vi "tracking1.vi"(6 "lane keep":bool, 10 "xbody":dbl, 11 "xt":dbl) -> (3 "handle":dbl=-3.32529799262397, 5 "Numeric":i32)   [LabVIEW 2015]
uses:
  G_PATH.vi
  G_VEH.vi
  G_NAV.vi
  G_SEN.vi
panel:
  out "v250":dbl[](array[numeric]) format="%.2f"
  in  "gain":dbl=0.7000000000000001
  in  "x":dbl=10.0
  in  "y":dbl=42.0
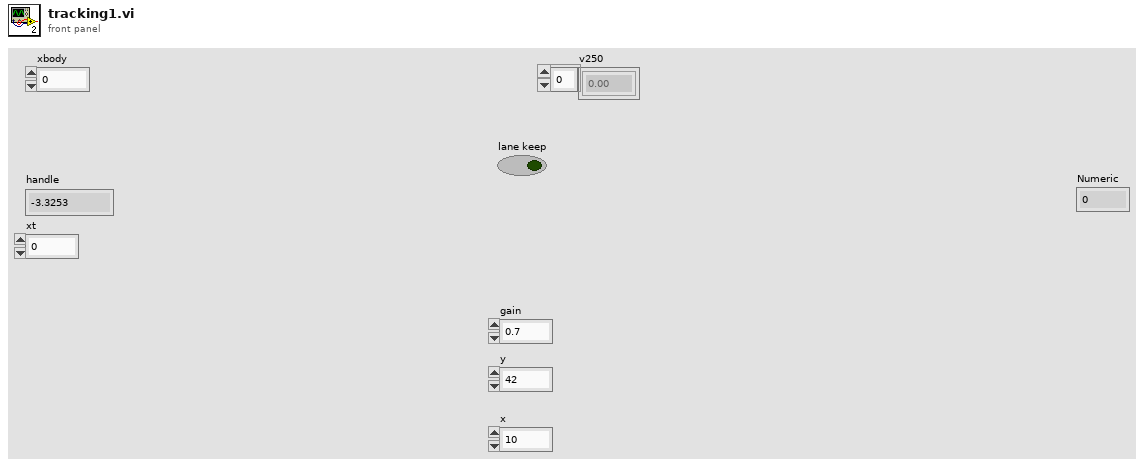
[diagram p1: front panel]
types:
  T1 = cluster{"idx":i32, "x":dbl, "y":dbl, "h":dbl, "x_path":dbl}
  T2 = cluster{"Steer_input":dbl, "Steer_output":dbl, "VS_des":dbl, "VS_can":dbl, "heading":dbl, "auto":bool, "run":bool, "x":dbl, "y":dbl}
  T3 = cluster{"GPSTime":dbl, "attitude[2]":dbl, "lcc[0]":dbl, "lcc[1]":dbl, "heading_GPS":dbl}
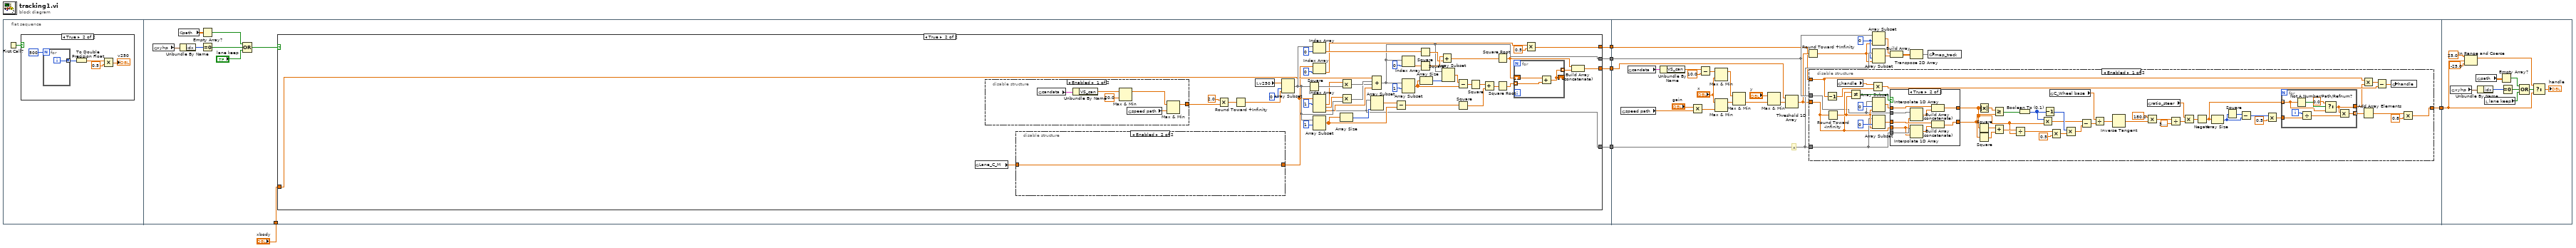
[diagram p0: block diagram]
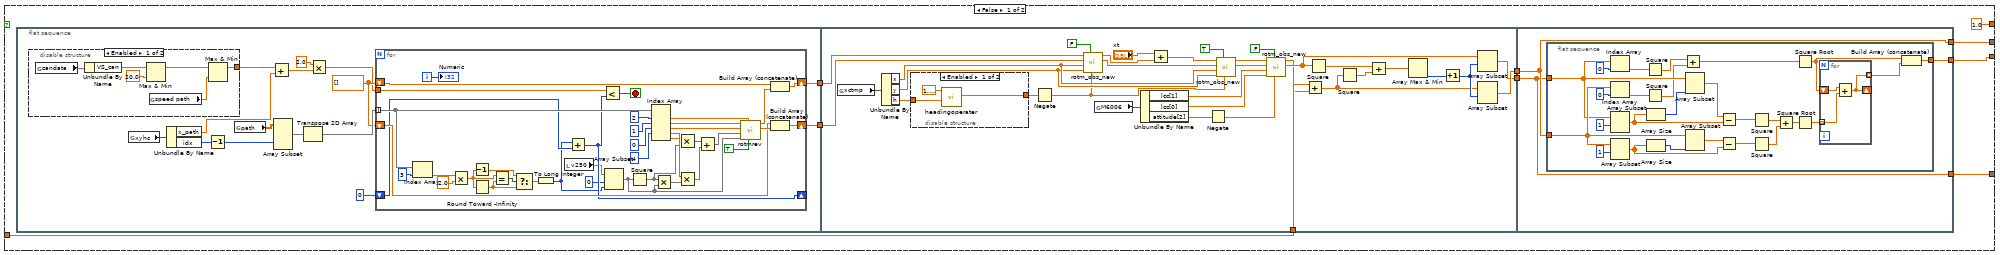
[diagram p3: hidden frame]
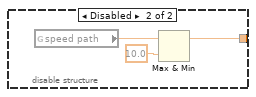
[diagram p4: hidden frame]
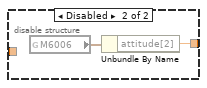
[diagram p5: hidden frame]
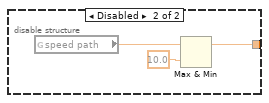
[diagram p6: hidden frame]
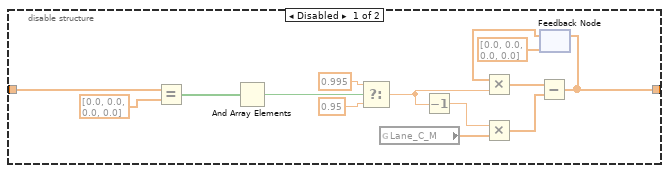
[diagram p7: hidden frame]
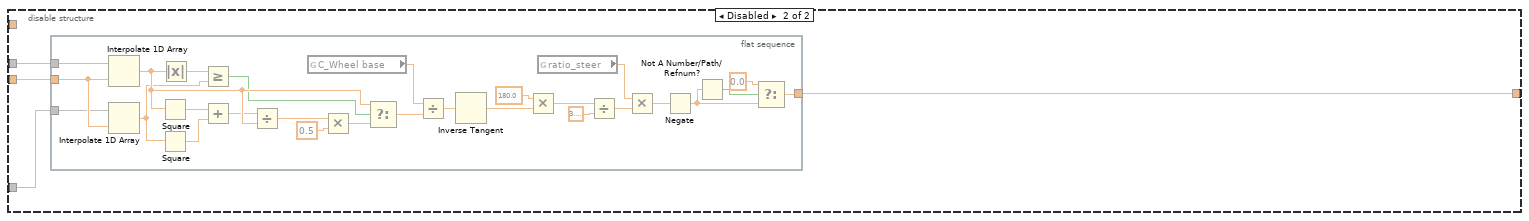
[diagram p9: hidden frame]
diagram:
  n1 = flat-sequence {
    tunnel: [w25] -> w6
    tunnel: [w24] -> w5
    tunnel: [w23] -> w4
    tunnel: "xbody" -> [w15]
    tunnel: [w14] -> w1
    tunnel: w6 -> [w262]
    tunnel: w5 -> [w252]
    tunnel: w4 -> [w251]
    tunnel: [w248] -> w3
    tunnel: w1 -> [w245]
    tunnel: w3 -> [w366]
    frame #0 {
      n2 = First Call?() -> (First Call?: T/F=w7:bool)
      n3 = case shown="True" w7 {
        frame False {
        }
        frame True {
          n4 = for {
            N: 500 -> [_]
            tunnel: [w13] -> w9 mode=indexing
            i -> [w13]
          }
          n5 = To Double Precision Float(number=w9) -> (double precision float=w10:dbl[])
          n6 = Multiply(x=w10, y=0.5 ("x")) -> (x*y=→"v250":dbl[])
        }
      }
    }
    frame #1 {
      n7 = global read "G_VEH.vi" "xyhp"() -> (w21:T1)
      n8 = global read "G_PATH.vi" "path"() -> (w18:dbl[][])
      n9 = Unbundle By Name(w21) -> ("idx"=w20:i32)
      n10 = Empty Array?(array=w18) -> (empty?=w17:bool)
      n11 = Equal To 0?(x=w20) -> (x = 0?=w19:bool)
      n12 = Compound Arithmetic op=OR(w17, w19, "lane keep") -> (w16:bool)
      n13 = case shown="True" w16 {
        tunnel: [w30 w204] -> w25
        tunnel: [w29 w180] -> w24
        tunnel: [w28 w174] -> w23
        tunnel: w15 -> [w27 w173]
        tunnel: [1.0 w168] -> w14
        frame False {
          n14 = flat-sequence {
            tunnel: [w42] -> w34
            tunnel: [w41] -> w33
            tunnel: [w124] -> w32
            tunnel: [w123] -> w31
            tunnel: w34 -> [w126]
            tunnel: w33 -> [w125]
            tunnel: w27 -> [w100]
            tunnel: w32 -> [w137]
            tunnel: w31 -> [w136]
            tunnel: [w138] -> w30
            tunnel: [w137] -> w29
            tunnel: [w136] -> w28
            frame #0 {
              w43 = dbl[] []
              n15 = disable-structure shown="Enabled" {
                disable-tunnel: [w50 w56] -> w35
                frame Enabled {
                  n16 = global read "G_VEH.vi" "candata"() -> (w55:T2)
                  n17 = Unbundle By Name(w55) -> ("VS_can"=w54:dbl)
                  n18 = Max & Min(x=w54, y=20.0) -> (max(x,y)=w52:dbl)  [unwired: 1 out]
                  n19 = global read "G_VEH.vi" "speed path"() -> (w51:dbl)
                  n20 = Max & Min(x=w52, y=w51) -> (max(x,y)=w50:dbl)  [unwired: 1 out]
                }
                frame Disabled {
                  n21 = global read "G_VEH.vi" "speed path"() -> (w58:dbl)
                  n22 = Max & Min(x=w58, y=10.0) -> (max(x,y)=w56:dbl)  [unwired: 1 out]
                }
              }
              n23 = global read "G_VEH.vi" "xyhc"() -> (w49:T1)
              n24 = Unbundle By Name(w49) -> ("x_path"=w36:dbl, "idx"=w48:i32)
              n25 = Decrement(x=w48) -> (x-1=w47:i32)
              n26 = global read "G_PATH.vi" "path"() -> (w46:dbl[][])
              n27 = Add(x=w35, y=w36) -> (x+y=w40:dbl)
              n28 = Array Subset(array=w46, index (col)=w47) -> (w45:dbl[][])  [unwired: 3 in]
              n29 = Transpose 2D Array(2D array=w45) -> (transposed array=w44:dbl[][])
              n30 = Multiply(x=2.0, y=w40) -> (x*y=w38:dbl)
              n31 = for {
                tunnel: w44 -> [w74] mode=indexing
                shift-right: [w72] -> w42
                shift-left: w43 -> [w71]
                shift-right: [w69] -> w41
                shift-left: w43 -> [w68]
                tunnel: w38 -> [w66]
                shift-right: [w65] -> _
                shift-left: 0 -> [w67]
                i -> [w64]
                stop <- w63 stop-if-true
                n32 = Index Array(array=w74, index=3) -> (element=w96:dbl)
                n33 = Multiply(x=w96, y=2.0) -> (x*y=w94:dbl)
                n34 = Decrement(x=w94) -> (x-1=w92:dbl)
                n35 = Round Toward -Infinity(1:w94) -> (0:w91:dbl)
                n36 = Equal?(x=w94, y=w91) -> (x = y?=w93:bool)
                n37 = Select(t=w92, s=w93, f=w91) -> (s? t:f=w90:dbl)
                n38 = To Long Integer(number=w90) -> (32bit integer=w60:i32)
                n39 = local read "v250"() -> (w62:dbl[])
                n40 = Add(x=w60, y=w67) -> (x+y=w65:i32)
                n41 = Less?(x=w66, y=w65) -> (x < y?=w63:bool)
                n42 = Array Subset(array=w62, index=0, length=w60) -> (w59:dbl[])
                n43 = Square(x=w59) -> (x^2=w77:dbl[])
                n44 = Index Array(array=w74, index #1=2 ("index"), index #2=1 ("index"), index #3=0 ("index"), index #4=4 ("index")) -> (element #1=w86:dbl, element #2=w87:dbl, element #3=w88:dbl, element #4=w78:dbl, element #5=w76:dbl)  [unwired: 1 in]
                n45 = Multiply(x=w77, y=w59) -> (x*y=w79:dbl[])
                n46 = Multiply(x=w76, y=w77) -> (x*y=w80:dbl[])
                n47 = Multiply(x=w78, y=w79) -> (x*y=w81:dbl[])
                n48 = Add(x=w80, y=w81) -> (x+y=w82:dbl[])
                n49 = call "rotmrev.vi"("reverse"=TRUE, "angle[rad]"=w86, "x"=w59, "y"=w82, "x0"=w88, "y0"=w87) -> ("y"=w70:dbl[], "x"=w73:dbl[])  [unwired: 4 in]
                n50 = Build Array (concatenate)(w71, w73) -> (w72:dbl[])
                n51 = Build Array (concatenate)(w68, w70) -> (w69:dbl[])
                "Numeric" <- w64
              }
            }
            frame #1 {
              n52 = global read "G_VEH.vi" "xctmp"() -> (w129:T1)
              n53 = Unbundle By Name(w129) -> ("x"=w112:dbl, "y"=w111:dbl, "h"=w128:dbl)
              n54 = disable-structure shown="Enabled" {
                disable-tunnel: w128 -> [w132 _]
                disable-tunnel: [w131 w134] -> w120
                frame Enabled {
                  n55 = call "headingoperater.vi"("h1"=w132, "h2"=1.5707963267948966) -> ("h2-h1"=w131:dbl)  [unwired: 8 in, 1 out]
                }
                frame Disabled {
                  n56 = global read "G_NAV.vi" "M6006"() -> (w135:T3)
                  n57 = Unbundle By Name(w135) -> ("attitude[2]"=w134:dbl)
                }
              }
              n58 = Negate(x=w120) -> (-x=w110:dbl)
              n59 = call "rotm_obs_new.vi"("angle[rad]"=w110, "reverse"=FALSE, "y0"=w111, "x0"=w112, "y"=w125, "x"=w126) -> ("rot*(y-y0) 2"=w114:dbl[], "rot*(x-x0)"=w119:dbl[])  [unwired: 2 in, 2 out]
              n60 = global read "G_NAV.vi" "M6006"() -> (w107:T3)
              n61 = Unbundle By Name(w107) -> ("lcc[1]"=w106:dbl, "lcc[0]"=w105:dbl, "attitude[2]"=w102:dbl)
              n62 = Add(x="xt", y=w119) -> (x+y=w115:dbl[])
              n63 = Negate(x=w102) -> (-x=w101:dbl)
              n64 = call "rotm_obs_new.vi"("angle[rad]"=w110, "reverse"=TRUE, "y0"=w111, "x0"=w112, "y"=w114, "x"=w115) -> ("rot*(y-y0) 2"=w108:dbl[], "rot*(x-x0)"=w109:dbl[])  [unwired: 2 in, 2 out]
              n65 = call "rotm_obs_new.vi"("angle[rad]"=w101, "reverse"=FALSE, "y0"=w105, "x0"=w106, "y"=w108, "x"=w109) -> ("rot*(y-y0) 2"=w103:dbl[], "rot*(x-x0)"=w98:dbl[])  [unwired: 2 in, 2 out]
              n66 = Add(x=w100, y=w98) -> (x+y=w99:dbl[])
              n67 = Square(x=w103) -> (x^2=w117:dbl[])
              n68 = Square(x=w99) -> (x^2=w116:dbl[])
              n69 = Add(x=w117, y=w116) -> (x+y=w127:dbl[])
              n70 = Array Max & Min(array=w127) -> (min index (indices)=w122:i32)  [unwired: 3 out]
              n71 = Increment(x=w122) -> (x+1=w121:i32)
              n72 = Array Subset(array=w103, index=w121) -> (w123:dbl[])  [unwired: 1 in]
              n73 = Array Subset(array=w99, index=w121) -> (w124:dbl[])  [unwired: 1 in]
            }
            frame #2 {
              n74 = flat-sequence {
                tunnel: [w145] -> w138
                tunnel: w137 -> [w144]
                tunnel: w136 -> [w143]
                frame #0 {
                  n75 = Index Array(array=w143, index=0) -> (element=w148:dbl)
                  n76 = Index Array(array=w144, index=0) -> (element=w149:dbl)
                  n77 = Array Subset(array=w143, index=1) -> (w158:dbl[])  [unwired: 1 in]
                  n78 = Array Subset(array=w144, index=1) -> (w161:dbl[])  [unwired: 1 in]
                  n79 = Square(x=w148) -> (x^2=w140:dbl)
                  n80 = Square(x=w149) -> (x^2=w139:dbl)
                  n81 = Array Size(array=w158) -> (size(s)=w156:i32)
                  n82 = Array Size(array=w161) -> (size(s)=w163:i32)
                  n83 = Add(x=w140, y=w139) -> (x+y=w147:dbl)
                  n84 = Array Subset(array=w143, length=w156) -> (w157:dbl[])  [unwired: 1 in]
                  n85 = Array Subset(array=w144, length=w163) -> (w162:dbl[])  [unwired: 1 in]
                  n86 = Subtract(x=w157, y=w158) -> (x-y=w159:dbl[])
                  n87 = Subtract(x=w162, y=w161) -> (x-y=w160:dbl[])
                  n88 = Square(x=w159) -> (x^2=w141:dbl[])
                  n89 = Square(x=w160) -> (x^2=w142:dbl[])
                  n90 = Add(x=w141, y=w142) -> (x+y=w153:dbl[])
                  n91 = Square Root(x=w147) -> (sqrt(x)=w146:dbl)
                  n92 = Square Root(x=w153) -> (sqrt(x)=w152:dbl[])
                  n93 = for {
                    tunnel: w152 -> [w166] mode=indexing
                    shift-right: [w165] -> _
                    shift-left: w146 -> [w167]
                    tunnel: [w165] -> w154 mode=indexing
                    n94 = Add(x=w167, y=w166) -> (x+y=w165:dbl)
                  }
                  n95 = Build Array (concatenate)(w146, w154) -> (w145:dbl[])
                }
              }
            }
          }
        }
        frame True {
          n96 = global read "G_SEN.vi" "Lane_C_M"() -> (w179:dbl[])
          n97 = disable-structure shown="Enabled" {
            disable-tunnel: [w214 w220] -> w178
            frame Enabled {
              n98 = global read "G_VEH.vi" "candata"() -> (w219:T2)
              n99 = Unbundle By Name(w219) -> ("VS_can"=w218:dbl)
              n100 = Max & Min(x=w218, y=20.0) -> (max(x,y)=w216:dbl)  [unwired: 1 out]
              n101 = global read "G_VEH.vi" "speed path"() -> (w215:dbl)
              n102 = Max & Min(x=w216, y=w215) -> (max(x,y)=w214:dbl)  [unwired: 1 out]
            }
            frame Disabled {
              n103 = global read "G_VEH.vi" "speed path"() -> (w222:dbl)
              n104 = Max & Min(x=w222, y=10.0) -> (max(x,y)=w220:dbl)  [unwired: 1 out]
            }
          }
          n105 = disable-structure shown="Enabled" {
            disable-tunnel: [w233 w237] -> w172
            disable-tunnel: w179 -> [w228 w237]
            frame Disabled {
              n106 = Equal?(x=w228, y=dbl[] [0.0, 0.0, 0.0, 0.0] ("Lane_C_M")) -> (x = y?=w227:bool[])
              n107 = And Array Elements(Boolean array=w227) -> (logical AND=w226:bool)
              n108 = Select(t=0.995, s=w226, f=0.95 ("filter")) -> (s? t:f=w225:dbl)
              n109 = global read "G_SEN.vi" "Lane_C_M"() -> (w230:dbl[])
              n110 = Decrement(x=w225) -> (x-1=w231:dbl)
              n111 = Multiply(x=w231, y=w230) -> (x*y=w236:dbl[])
              n112 = feedback #1(dbl[] [0.0, 0.0, 0.0, 0.0] ("Lane_C_M")) -> (w235:dbl[])
              n113 = Multiply(x=w235, y=w225) -> (x*y=w234:dbl[])
              n114 = Subtract(x=w234, y=w236) -> (x-y=w233:dbl[])
              n115 = feedback-in #1(w233) -> ()
            }
            frame Enabled {
            }
          }
          n116 = Multiply(x=2.0, y=w178) -> (x*y=w212:dbl)
          n117 = Round Toward +Infinity(x=w212) -> (ceil(x): smallest int >= x=w176:dbl)
          n118 = local read "v250"() -> (w177:dbl[])
          n119 = Array Subset(array=w177, index=0, length=w176) -> (w174:dbl[])
          n120 = Square(x=w174) -> (x^2=w210:dbl[])
          n121 = Index Array(array=w174, index=0) -> (element=w185:dbl)
          n122 = Index Array(array=w172, index=0) -> (element=w169:dbl)
          n123 = Index Array(array=w172, index #1=1 ("index")) -> (element #1=w209:dbl, element #2=w208:dbl, element #3=w205:dbl)  [unwired: 2 in]
          n124 = Array Subset(array=w174, index=1) -> (w197:dbl[])  [unwired: 1 in]
          n125 = Multiply(x=w209, y=w210) -> (x*y=w207:dbl[])
          n126 = Multiply(x=w208, y=w174) -> (x*y=w206:dbl[])
          n127 = Array Size(array=w197) -> (size(s)=w195:i32)
          n128 = Array Subset(array=w174, length=w195) -> (w196:dbl[])  [unwired: 1 in]
          n129 = Compound Arithmetic op=ADD(w173, w207, w206, w205) -> (w180:dbl[])
          n130 = Subtract(x=w196, y=w197) -> (x-y=w198:dbl[])
          n131 = Index Array(array=w180, index=0) -> (element=w186:dbl)
          n132 = Array Subset(array=w180, index=1) -> (w200:dbl[])  [unwired: 1 in]
          n133 = Square(x=w185) -> (x^2=w182:dbl)
          n134 = Square(x=w186) -> (x^2=w183:dbl)
          n135 = Array Size(array=w200) -> (size(s)=w202:i32)
          n136 = Add(x=w183, y=w182) -> (x+y=w184:dbl)
          n137 = Array Subset(array=w180, length=w202) -> (w201:dbl[])  [unwired: 1 in]
          n138 = Square(x=w198) -> (x^2=w192:dbl[])
          n139 = Subtract(x=w201, y=w200) -> (x-y=w199:dbl[])
          n140 = Square(x=w199) -> (x^2=w193:dbl[])
          n141 = Add(x=w193, y=w192) -> (x+y=w190:dbl[])
          n142 = Square Root(x=w184) -> (sqrt(x)=w181:dbl)
          n143 = Square Root(x=w190) -> (sqrt(x)=w189:dbl[])
          n144 = for {
            tunnel: w189 -> [w239] mode=indexing
            shift-right: [w238] -> _
            shift-left: w181 -> [w240]
            tunnel: [w238] -> w191 mode=indexing
            n145 = Add(x=w240, y=w239) -> (x+y=w238:dbl)
          }
          n146 = Multiply(x=w169, y=0.5 ("x")) -> (x*y=w168:dbl)
          n147 = Build Array (concatenate)(w181, w191) -> (w204:dbl[])
        }
      }
    }
    frame #2 {
      w246 = 0 ("index")
      # "x"
      n148 = global read "G_VEH.vi" "speed path"() -> (w256:dbl)
      n149 = global read "G_VEH.vi" "candata"() -> (w261:T2)
      n150 = Unbundle By Name(w261) -> ("VS_can"=w254:dbl)
      n151 = Multiply(x="gain", y=w256) -> (x*y=w242:dbl)
      n152 = Subtract(x=w254, y=10.0) -> (x-y=w244:dbl)
      n153 = Max & Min(x=w244, y="x") -> (max(x,y)=w259:dbl)  [unwired: 1 out]
      n154 = Max & Min(x="x", y=w242) -> (max(x,y)=w258:dbl)  [unwired: 1 out]
      n155 = Max & Min(x=w259, y=w258) -> (min(x,y)=w257:dbl)  [unwired: 1 out]
      n156 = Max & Min(x="y", y=w257) -> (min(x,y)=w263:dbl)  [unwired: 1 out]
      n157 = Threshold 1D Array(2:w263, 3:w262) -> (0:w247:dbl)  [unwired: 1 in]
      n158 = Round Toward +Infinity(x=w247) -> (ceil(x): smallest int >= x=w241:dbl)
      n159 = disable-structure shown="Enabled" {
        disable-tunnel: w252 -> [w274 w338]
        disable-tunnel: w251 -> [w279 w337]
        disable-tunnel: [w283 w335] -> w248
        disable-tunnel: w247 -> [w278 w336]
        disable-tunnel: w245 -> [w266 _]
        frame Enabled {
          n160 = Decrement(x=w266) -> (x-1=w272:dbl)
          n161 = Round Toward -Infinity(1:w278) -> (0:w281:dbl)
          n162 = global read "G_VEH.vi" "handle"() -> (w271:dbl)
          n163 = Not Equal?(x=w278, y=w281) -> (x != y?=w280:bool)
          n164 = Multiply(x=w271, y=w272) -> (x*y=w269:dbl)
          n165 = Array Subset(array=w274, index=0, length=w281) -> (w275:dbl[])
          n166 = Array Subset(array=w279, index=0, length=w281) -> (w277:dbl[])
          n167 = case shown="True" w280 {
            tunnel: w279 -> [_ w326]
            tunnel: w278 -> [_ w319]
            tunnel: w277 -> [w317 w325]
            tunnel: [w317 w323] -> w276
            tunnel: w275 -> [w316 w321]
            tunnel: w274 -> [_ w320]
            tunnel: [w316 w318] -> w273
            frame False {
            }
            frame True {
              n168 = Interpolate 1D Array(1:w319, 2:w320) -> (0:w322:dbl)
              n169 = Interpolate 1D Array(1:w319, 2:w326) -> (0:w324:dbl)
              n170 = Build Array (concatenate)(w321, w322) -> (w318:dbl[])
              n171 = Build Array (concatenate)(w325, w324) -> (w323:dbl[])
            }
          }
          n172 = Square(x=w273) -> (x^2=w301:dbl[])
          n173 = Square(x=w276) -> (x^2=w302:dbl[])
          n174 = Absolute Value(x=w273) -> (abs(x)=w300:dbl[])
          n175 = Greater Or Equal?(x=w300, y=w276) -> (x >= y?=w299:bool[])
          n176 = Add(x=w301, y=w302) -> (x+y=w303:dbl[])
          n177 = Divide(x=w303, y=w273) -> (x/y=w304:dbl[])
          n178 = Boolean To (0,1)(Boolean=w299) -> (0, 1=w298:i16[])
          n179 = Multiply(x=w298, y=w273) -> (x*y=w294:dbl[])
          n180 = Decrement(x=w298) -> (x-1=w296:i16[])
          n181 = global read "G_VEH.vi" "C_Wheel base"() -> (w306:dbl)
          n182 = Multiply(x=w304, y=0.5) -> (x*y=w297:dbl[])
          n183 = Multiply(x=w296, y=w297) -> (x*y=w295:dbl[])
          n184 = Subtract(x=w294, y=w295) -> (x-y=w293:dbl[])
          n185 = Divide(x=w306, y=w293) -> (x/y=w307:dbl[])
          n186 = Inverse Tangent(1:w307) -> (0:w309:dbl[])
          n187 = Multiply(x=180.0 ("y"), y=w309) -> (x*y=w310:dbl[])
          n188 = global read "G_VEH.vi" "ratio_steer"() -> (w313:dbl)
          n189 = Divide(x=w310, y=3.141592653589793) -> (x/y=w312:dbl[])
          n190 = Multiply(x=w313, y=w312) -> (x*y=w314:dbl[])
          n191 = Negate(x=w314) -> (-x=w290:dbl[])
          n192 = Array Size(array=w290) -> (size(s)=w288:i32)
          n193 = Square(x=w288) -> (x^2=w289:i32)
          n194 = Subtract(x=w289, y=w288) -> (x-y=w287:i32)
          n195 = Multiply(x=w287, y=0.5) -> (x*y=w285:dbl)
          n196 = for {
            tunnel: w290 -> [w332] mode=indexing
            tunnel: [w331] -> w315 mode=indexing
            tunnel: w285 -> [w329]
            tunnel: [w327] -> w267
            i -> [w330]
            n197 = Not A Number/Path/Refnum?(number/path/refnum=w332) -> (NaN/Path/Refnum?=w334:bool)
            n198 = Divide(x=w330, y=w329) -> (x/y=w328:dbl)
            n199 = Select(t=0.0, s=w334, f=w332) -> (s? t:f=w327:dbl)
            n200 = Multiply(x=w327, y=w328) -> (x*y=w331:dbl)
          }
          n201 = Multiply(x=w266, y=w267) -> (x*y=w270:dbl)
          n202 = Add Array Elements(numeric array=w315) -> (sum=w284:dbl)
          n203 = Subtract(x=w270, y=w269) -> (x-y=w268:dbl)
          n204 = global write "G_VEH.vi" "handle"(w268) -> ()
          n205 = Multiply(x=w284, y=0.8) -> (x*y=w283:dbl)
        }
        frame Disabled {
          n206 = flat-sequence {
            tunnel: w336 -> [w363]
            tunnel: w338 -> [w362]
            tunnel: w337 -> [w361]
            tunnel: [w339] -> w335
            frame #0 {
              n207 = Interpolate 1D Array(1:w363, 2:w362) -> (0:w365:dbl)
              n208 = Interpolate 1D Array(1:w363, 2:w361) -> (0:w364:dbl)
              n209 = Square(x=w365) -> (x^2=w345:dbl)
              n210 = Square(x=w364) -> (x^2=w346:dbl)
              n211 = Absolute Value(x=w365) -> (abs(x)=w344:dbl)
              n212 = Greater Or Equal?(x=w344, y=w364) -> (x >= y?=w343:bool)
              n213 = Add(x=w345, y=w346) -> (x+y=w347:dbl)
              n214 = Divide(x=w347, y=w365) -> (x/y=w348:dbl)
              n215 = global read "G_VEH.vi" "C_Wheel base"() -> (w351:dbl)
              n216 = Multiply(x=w348, y=0.5) -> (x*y=w350:dbl)
              n217 = Select(t=w365, s=w343, f=w350) -> (s? t:f=w352:dbl)
              n218 = Divide(x=w351, y=w352) -> (x/y=w353:dbl)
              n219 = Inverse Tangent(1:w353) -> (0:w355:dbl)
              n220 = Multiply(x=180.0 ("y"), y=w355) -> (x*y=w356:dbl)
              n221 = global read "G_VEH.vi" "ratio_steer"() -> (w359:dbl)
              n222 = Divide(x=w356, y=3.141592653589793) -> (x/y=w358:dbl)
              n223 = Multiply(x=w359, y=w358) -> (x*y=w360:dbl)
              n224 = Negate(x=w360) -> (-x=w340:dbl)
              n225 = Not A Number/Path/Refnum?(number/path/refnum=w340) -> (NaN/Path/Refnum?=w342:bool)
              n226 = Select(t=0.0, s=w342, f=w340) -> (s? t:f=w339:dbl)
            }
          }
        }
      }
      n227 = Array Subset(array=w252, index=w246, length=w241) -> (w250:dbl[])
      n228 = Array Subset(array=w251, index=w246, length=w241) -> (w249:dbl[])
      n229 = Build Array(w250, w249) -> (w265:dbl[][])
      n230 = Transpose 2D Array(2D array=w265) -> (transposed array=w264:dbl[][])
      n231 = global write "G_PATH.vi" "map_track"(w264) -> ()
    }
    frame #3 {
      n232 = global read "G_VEH.vi" "xyhp"() -> (w372:T1)
      n233 = In Range and Coerce(upper limit=25.0, x=w366, lower limit=-25.0) -> (coerced(x)=w375:dbl)  [unwired: 1 out]
      n234 = global read "G_PATH.vi" "path"() -> (w369:dbl[][])
      n235 = Unbundle By Name(w372) -> ("idx"=w371:i32)
      n236 = local read "lane keep"() -> (w377:bool)
      n237 = Empty Array?(array=w369) -> (empty?=w368:bool)
      n238 = Equal To 0?(x=w371) -> (x = 0?=w370:bool)
      n239 = Compound Arithmetic op=OR(w368, w370, w377) -> (w376:bool)
      n240 = Select(t=w375, s=w376, f=w366) -> (s? t:f=→"handle":dbl)
    }
  }
